vi "CANopen Node Guarding.vi"() -> ()   [LabVIEW 2016]
doc: "This example demonstrates how to read a CANopen node guarding object."
uses:
  <vilib>/userdefined/High Color/nirio_resource_hc.ctl
  <vilib>/Platform/TimedLoop/XDataNode/timing_clust.ctl
  <vilib>/Platform/TimedLoop/XDataNode/nitl_modes.ctl
  <vilib>/Platform/TimedLoop/XDataNode/wakeup.ctl
  <vilib>/FPGAPlugInAG/cRIO-9033/niLvFpga_Open_cRIO-9033.vi
  <vilib>/rvi/interface/common/dynamic/niFpgaDynamicAddResources.vi
  <vilib>/CANopenLib/CANOPEN.llb/CANopen Interface Create.vi
  <vilib>/CANopenLib/CANOPEN.llb/CANopen SDO Create.vi
  <vilib>/CANopenLib/CANOPEN.llb/CANopen SDO Write [U16].vi
  <vilib>/CANopenLib/CANOPEN.llb/CANopen SDO Write [U8].vi
  <vilib>/CANopenLib/CANOPEN.llb/CANopen SDO Close.vi
  <vilib>/CANopenLib/CANOPEN.llb/CANopen Node Guarding Create.vi
  <vilib>/CANopenLib/CANOPEN.llb/CANopen Node Guarding Start.vi
  <vilib>/CANopenLib/CANOPEN.llb/CANopen Node Guarding State Read.vi
  <vilib>/CANopenLib/CANOPEN.llb/CANopen Node Guarding Close.vi
  <vilib>/CANopenLib/CANOPEN.llb/CANopen Interface Close.vi
  <vilib>/FPGAPlugInAG/Dynamic/niLvFpga_Close_Dynamic.vi
  <vilib>/rvi/interface/nirviOpenFPGA/nirviOpenFPGA.xnode
  FPGA Bitfiles/project_FPGATarget_MainFPGA_S9ZLErdeBuw.lvbitx
  FPGA/MainFPGA.vi
  <vilib>/Platform/TimedLoop/XDataNode/XDataNode.xnode
  <vilib>/rvi/interface/nirviCloseFPGA/nirviCloseFPGA.xnode
  <vilib>/Platform/TimedLoop/XDataNode/XDNodeRunTimeDep.lvlib
panel:
  in  "error in":errorcluster
  out "timestamp":timestamp
  out "state":u16(ring)=1 items=["unknown"=1, "boot-up"=0, "stopped"=4, "operational"=5, "pre-operational"=127, "connection lost"=128]
  in  "stop":bool
  in  "period (ms)":i64=10
  in  "guard time (ms)":u16=5
  in  "node-ID":u8=1 min=1 max=127 step=1
  in  "baud rate":u32(ring)=2 items=["1 Mbit/s"=0, "800 kbit/s"=1, "500 kbit/s"=2, "250 kbit/s"=3, "125 kbit/s"=4, "50 kbit/s"=6, "20 kbit/s"=7, "10 kbit/s"=8]
  in  "CANopen interface":u32(ring) items=["CANopen01", "CANopen02", "CANopen03", "CANopen04", "CANopen05", "CANopen06", "CANopen07", "CANopen08", "CANopen09", "CANopen10", "CANopen11", "CANopen12", "CANopen13", "CANopen14", "CANopen15", "CANopen16", "CANopen17", "CANopen18", "CANopen19", "CANopen20", "CANopen21", "CANopen22", "CANopen23", "CANopen24", "CANopen25", "CANopen26", "CANopen27", "CANopen28", "CANopen29", "CANopen30", "CANopen31", "CANopen32"]
  # "Overview: This example demonstrates how to read a CANopen Node Guarding object.\nRequirements: Connect CANopen module with a slave device. \nInstructions:\n1. Specify the values of CANopen interface, baud rate of the CANopen interface, node-ID of the slave device and \n    guard time (ms) of Node Guarding object.\n2. Run this VI.\n3. Click STOP to stop the VI."
  # "Create CANopen interface and Node Guarding object"
  # "Read Node Guarding messages"
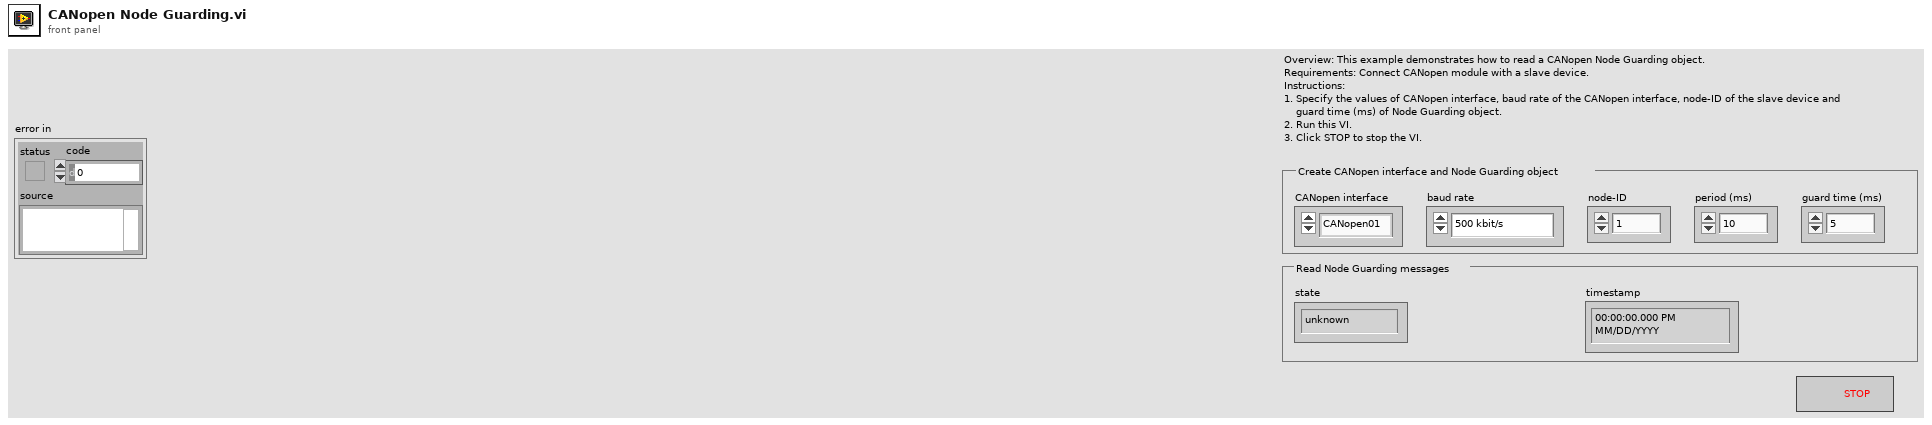
[diagram p1: front panel]
types:
  T1 = typedef "nirio_resource_hc.ctl" = tag
  T2 = typedef "XDNodeRunTimeDep.lvlib/timing_clust.ctl" = cluster{"Expected End [f-1]":u64, "Actual End [f-1]":u64, "Finished Late? [f-1]":bool, "Expected End [i-1]":u64, "Actual End [i-1]":u64, "Finished Late? [i-1]":bool, "Expected Start [i]":u64, "Actual Start [i]":u64, "Expected Start [f]":u64, "Actual Start [f]":u64, "Source Name":string, "Structure Name":string, "Period":i64, "Deadline":i64, "Offset":i64, "Start":i64, "Priority":i32, "Timeout":i32, "Mode":T3, "Wakeup Reason":T4, "Error":errorcluster, "Source Type":string, "Secondary Source Type":string, "Global End Time":u64, "Global Start Time":u64, "Frame Duration":u64, "Iteration Duration":u64, "Assigned CPU":i32, "I/O Scan Engine Mode":u32}
  T3 = typedef "XDNodeRunTimeDep.lvlib/nitl_modes.ctl" = enum32{"No Change", "Process missed periods, maintain original phase", "Discard missed periods, maintain original phase", "Process missed periods, ignore original phase", "Discard missed periods, ignore original phase"}
  T4 = typedef "XDNodeRunTimeDep.lvlib/wakeup.ctl" = enum32{"Normal", "Aborted", "Asynchronous wakeup", "Timing source error", "Timed loop error", "Timeout"}
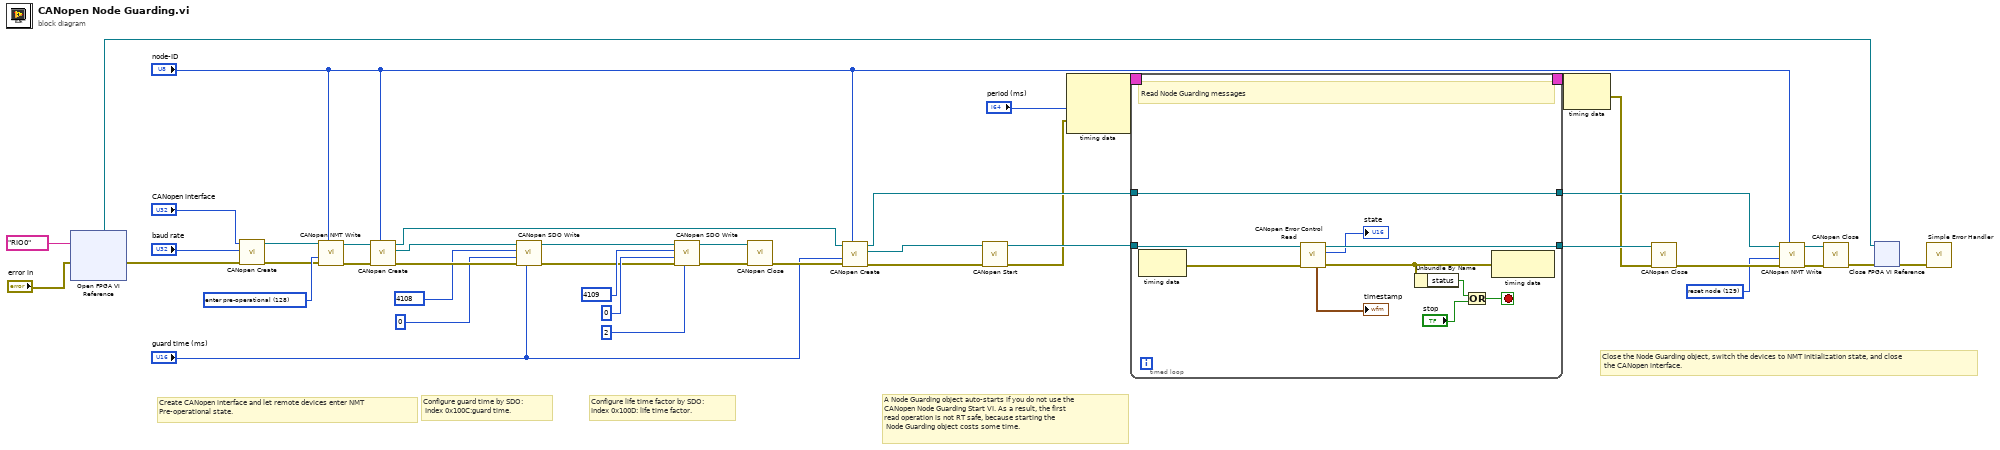
[diagram p0: block diagram]
diagram:
  w30 = u16 129 items=["start remote node"=1, "stop remote node"=2, "enter pre-operational"=128, "reset node"=129, "reset communication"=130] ("command")
  w39 = u16 128 items=["start remote node"=1, "stop remote node"=2, "enter pre-operational"=128, "reset node"=129, "reset communication"=130] ("command")
  # "A Node Guarding object auto-starts if you do not use the \nCANopen Node Guarding Start VI. As a result, the first \nread operation is not RT safe, because starting the\n Node Guarding object costs some time."
  # "Close the Node Guarding object, switch the devices to NMT Initialization state, and close\n the CANopen interface."
  # "Create CANopen interface and let remote devices enter NMT\nPre-operational state."
  # "Configure life time factor by SDO:\nIndex 0x100D: life time factor."
  # "Configure guard time by SDO:\n Index 0x100C:guard time."
  n1 = xnode ("Open FPGA VI Reference")("error in"="error in", "resource name"=T1 "RIO0") -> ("FPGA VI Reference Out"=w1:refnum<k20>, "error out"=w4:errorcluster)
  n2 = call-poly <vilib>:"CANopen Create.vi"("error in (no error)"=w4, "baud rate"="baud rate", "interface name"="CANopen interface") -> ("error out"=w38:errorcluster, "interface object out"=w37:refnum<k20>)  [unwired: 7 in]
  n3 = call <vilib>:"CANopen NMT Write.vi"("node-ID (0)"="node-ID", "error in (no error)"=w38, "command"=w39, "interface object in"=w37) -> ("error out"=w22:errorcluster, "interface object out"=w24:refnum<k20>)  [unwired: 6 in]
  n4 = call-poly <vilib>:"CANopen Create.vi"("node-ID"="node-ID", "error in (no error)"=w22, "interface object in"=w24) -> ("error out"=w27:errorcluster, "SDO object out"=w28:refnum<k20>, "interface object out"=w23:refnum<k20>)  [unwired: 6 in]
  n5 = call-poly <vilib>:"CANopen SDO Write.vi"("U16 data"="guard time (ms)", "error in (no error)"=w27, "object sub-index (0)"=u8 0, "object index"=u16 4108, "SDO object in"=w28) -> ("error out"=w17:errorcluster, "SDO object out"=w19:refnum<k20>)  [unwired: 4 in, 1 out]
  n6 = call-poly <vilib>:"CANopen SDO Write.vi"("U8 data"=u8 2, "error in (no error)"=w17, "object sub-index (0)"=u8 0, "object index"=u16 4109, "SDO object in"=w19) -> ("error out"=w16:errorcluster, "SDO object out"=w18:refnum<k20>)  [unwired: 4 in, 1 out]
  n7 = call-poly <vilib>:"CANopen Close.vi"("error in (no error)"=w16, "SDO object in"=w18) -> ("error out"=w15:errorcluster)  [unwired: 9 in]
  n8 = call-poly <vilib>:"CANopen Create.vi"("node-ID"="node-ID", "error in (no error)"=w15, "guard time [ms]"="guard time (ms)", "interface object in"=w23) -> ("error out"=w13:errorcluster, "node guarding object out"=w12:refnum<k20>, "interface object out"=w31:refnum<k20>)  [unwired: 5 in]
  n9 = call-poly <vilib>:"CANopen Start.vi"("error in (no error)"=w13, "node guarding object in"=w12) -> ("error out"=w10:errorcluster, "node guarding object out"=w35:refnum<k20>)  [unwired: 8 in]
  n10 = node-c288("period (ms)", w10) -> (w43:T2)  [unwired: 1 in]
  n11 = timed-loop {
    tunnel: w35 -> [w52]
    tunnel: [w51] -> w36
    tunnel: [w49] -> w32
    tunnel: w31 -> [w49]
    timing: w43 -> [_]
    timing-out: [_] -> w42
    stop <- w48 stop-if-true
    # "Read Node Guarding messages"
    n12 = node-c288() -> (w45:errorcluster)  [unwired: 1 in]
    n13 = call-poly <vilib>:"CANopen Error Control Read.vi"("error in (no error)"=w45, "node guarding object in"=w52) -> ("error out"=w44:errorcluster, "state"=→"state":u16, "node guarding object out"=w51:refnum<k20>, "timestamp"=→"timestamp":timestamp)  [unwired: 6 in]
    n14 = Unbundle By Name(w44) -> ("status"=w46:bool)
    n15 = Or(x=w46, y="stop") -> (x .or. y?=w48:bool)
    n16 = node-c288(w44) -> ()  [unwired: 1 out]
  }
  n17 = node-c288(w42) -> (w9:errorcluster)
  n18 = call-poly <vilib>:"CANopen Close.vi"("error in (no error)"=w9, "node guarding object in"=w36) -> ("error out"=w33:errorcluster)  [unwired: 9 in]
  n19 = call <vilib>:"CANopen NMT Write.vi"("node-ID (0)"="node-ID", "error in (no error)"=w33, "command"=w30, "interface object in"=w32) -> ("error out"=w34:errorcluster, "interface object out"=w29:refnum<k20>)  [unwired: 6 in]
  n20 = call-poly <vilib>:"CANopen Close.vi"("error in (no error)"=w34, "interface object in"=w29) -> ("error out"=w3:errorcluster)  [unwired: 9 in]
  n21 = xnode "Close FPGA VI Reference"("FPGA VI Reference In"=w1, "error in"=w3) -> ("error out"=w2:errorcluster)
  n22 = call <vilib>:"Simple Error Handler.vi"("error in (no error)"=w2) -> ()  [unwired: 4 in, 5 out]
